vi "ParseCommaList.vi"(11 "value":string) -> (3 "Array":string[](array[string]))   [LabVIEW 2017]
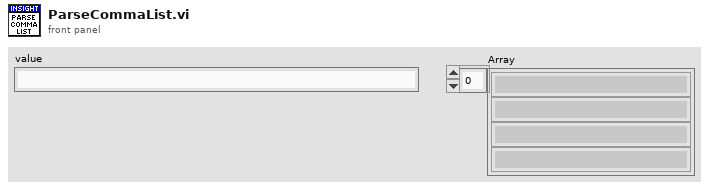
[diagram p1: front panel]
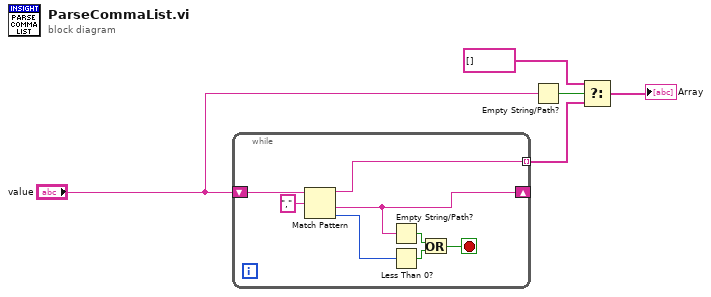
[diagram p0: block diagram]
diagram:
  n1 = while {
    shift-right: [w10] -> _
    shift-left: "value" -> [w13]
    tunnel: [w11] -> w5 mode=indexing
    stop <- w6 stop-if-true
    n2 = Match Pattern(string=w13, regular expression=",") -> (before substring=w11:string, after substring=w10:string, offset past match=w9:i32)  [unwired: 1 in, 1 out]
    n3 = Empty String/Path?(string/path=w10) -> (empty?=w7:bool)
    n4 = Less Than 0?(x=w9) -> (x < 0?=w8:bool)
    n5 = Or(x=w7, y=w8) -> (x .or. y?=w6:bool)
  }
  n6 = Empty String/Path?(string/path="value") -> (empty?=w3:bool)
  n7 = Select(t=string[] [], s=w3, f=w5) -> (s? t:f=→"Array":string[])
